vi "options.vi"(9 "server information":T1, 10 "application request in":T5, 11 "test responder in":refnum<class "test responder.lvclass">) -> (2 "application response out":T2, 3 "test responder out":refnum<class "test responder.lvclass">)   [LabVIEW 2013, in "test responder.lvclass"]
uses:
  test responder.lvclass
  HTTP server/http request.ctl
  HTTP server/http method.ctl
  HTTP headers/http header data.ctl
  HTTP server/http response.ctl
  HTTP server/http response packet type.ctl
  HTTP server/http server info.ctl
  HTTP responder/http responder.lvclass
  HTTP server/Basic HTTP server.lvclass
  HTTP headers/http headers.lvlib
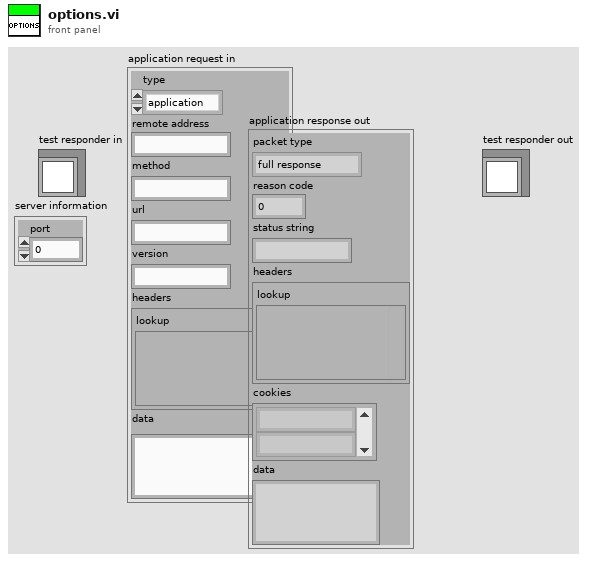
[diagram p1: front panel]
types:
  T1 = typedef "Basic HTTP server.lvclass/http server info.ctl" = cluster{"port":u16}
  T2 = typedef "Basic HTTP server.lvclass/http response.ctl" = cluster{"packet type":T3, "reason code":u16, "status string":string, "headers":T4, "cookies":string[], "data":string}
  T3 = typedef "Basic HTTP server.lvclass/http response packet type.ctl" = enum16{"full response", "header only", "data only", "last data", "raw output"}
  T4 = typedef "http headers.lvlib/http header data.ctl" = cluster{"lookup":variant}
  T5 = typedef "Basic HTTP server.lvclass/http request.ctl" = cluster{"type":T6, "remote address":string, "method":string, "url":string, "version":string, "headers":T4, "data":string}
  T6 = typedef "Basic HTTP server.lvclass/http method.ctl" = enum16{"application", "error", "upgrade", "expect"}
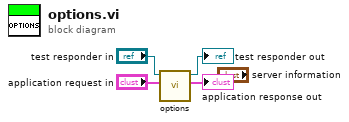
[diagram p0: block diagram]
diagram:
  n1 = call-parent "options.vi"("application request in"="application request in", "http responder in"="test responder in") -> ("application response out"=→"application response out":T2, "http responder out"=→"test responder out":refnum<class "test responder.lvclass">)  [unwired: 8 in]
